vi "gentec-SOLO-PE.set Wavelength.vi"(8 "error in (no error)":errorcluster, 10 "Wavelength [nm]":u32=1064, 11 "VISA Refnum in":refnum<visa-resource-name>) -> (0 "error out":errorcluster, 1 "Acknoledged?":bool, 2 "Error":string, 3 "VISA Refnum out":refnum<visa-resource-name>, 4 "Timeout":bool)   [LabVIEW 2014, in "gentec-SOLO-PE - Driver.lvlib"]
doc: "Sets the Wavelength in Nanometer."
uses:
  gentec-SOLO-PE - Driver.lvlib
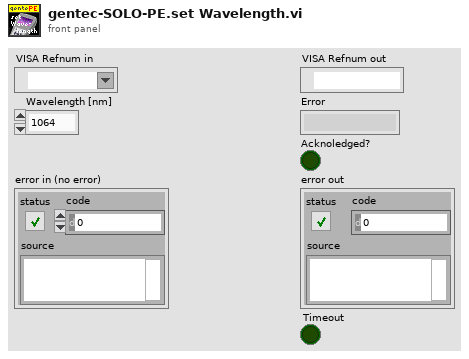
[diagram p1: front panel]
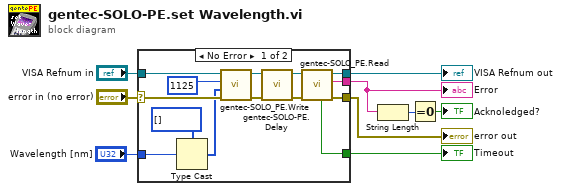
[diagram p0: block diagram]
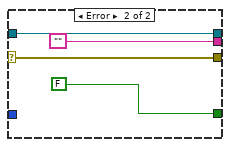
[diagram p2: hidden frame]
diagram:
  n1 = case shown="No Error" "error in (no error)" {
    selector: "error in (no error)" -> [w15 w26]
    tunnel: [w13 w26] -> w9
    tunnel: [w23 w27] -> w8
    tunnel: [w14 ""] -> w3
    tunnel: [w22 FALSE ("Timeout")] -> w7
    tunnel: "VISA Refnum in" -> [w17 w27]
    tunnel: "Wavelength [nm]" -> [w10 _]
    frame No Error {
      n2 = Type Cast(type=u32[] [], x=w10) -> (*(type *) &x=w11:u32[])
      n3 = call "gentec-SOLO_PE.Write.vi"("error in (no error)"=w15, "Parameters (Empty)"=w11, "Command Handle"=u16 1125, "VISA Refnum in"=w17) -> ("error out"=w20:errorcluster, "VISA Refnum out"=w18:refnum<visa-resource-name>)  [unwired: 6 in]
      n4 = call "gentec-SOLO-PE.Delay.vi"("error in (no error)"=w20, "VISA resource In"=w18) -> ("error out"=w21:errorcluster, "VISA resource Out"=w19:refnum<visa-resource-name>)  [unwired: 4 in]
      n5 = call "gentec-SOLO_PE.Read.vi"("error in (no error)"=w21, "VISA Refnum in"=w19) -> ("error out"=w13:errorcluster, "Error"=w14:string, "VISA Refnum out"=w23:refnum<visa-resource-name>, "Timeout"=w22:bool)  [unwired: 5 in, 1 out]
    }
    frame Error {
    }
  }
  "error out" <- w9
  "VISA Refnum out" <- w8
  "Error" <- w3
  "Timeout" <- w7
  n6 = String Length(string=w3) -> (length=w2:i32)
  n7 = Equal To 0?(x=w2) -> (x = 0?=→"Acknoledged?":bool)
